vi "Channel_Map_Global.vi"() -> ()   [LabVIEW 2021]
uses:
  Channel_Cluster.ctl
panel:
  out "Channels map":T1[](array[typedef])
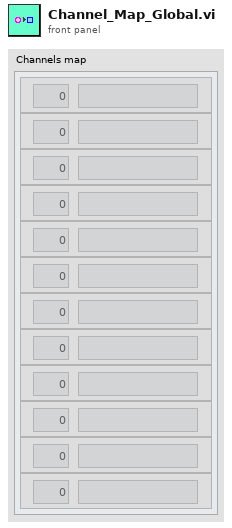
[diagram p1: front panel]
types:
  T1 = typedef "Channel_Cluster.ctl" = cluster{"Channel name":string, "Channel":u8}
diagram:
